vi "mini project.vi"() -> ()   [LabVIEW 2013]
panel:
  out "resulting string":string
  out "x":u8
  out "unsigned byte array":u8[](array[numeric])
  in  "String":string
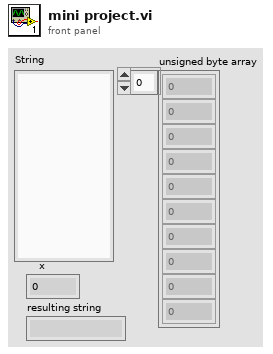
[diagram p1: front panel]
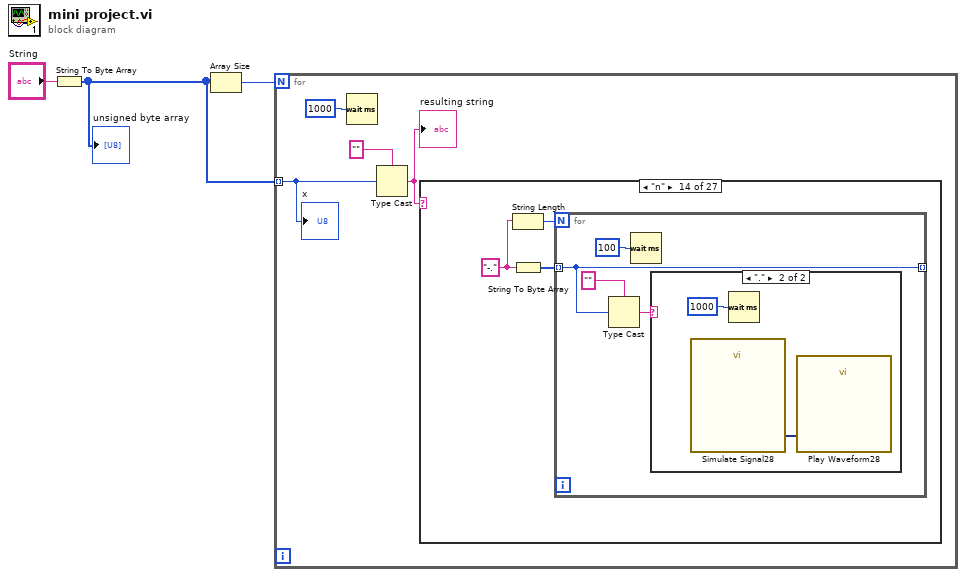
[diagram p0: block diagram]
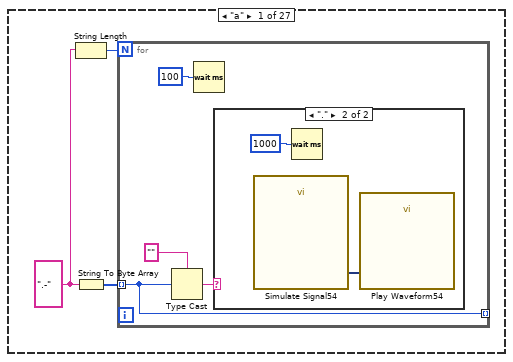
[diagram p2: hidden frame]
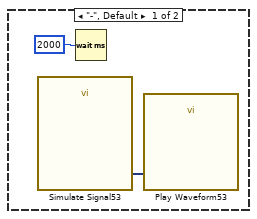
[diagram p3: hidden frame]
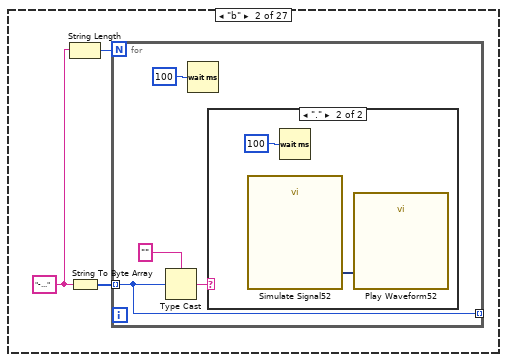
[diagram p4: hidden frame]
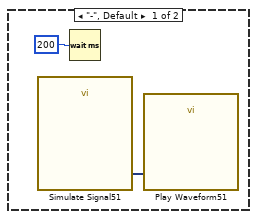
[diagram p5: hidden frame]
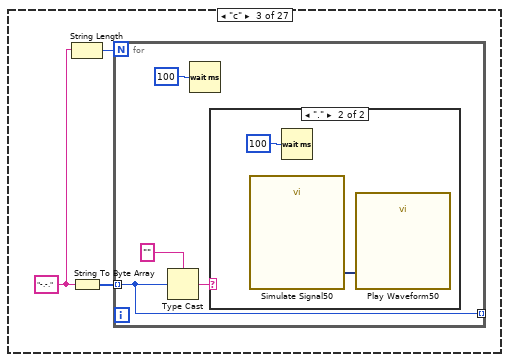
[diagram p6: hidden frame]
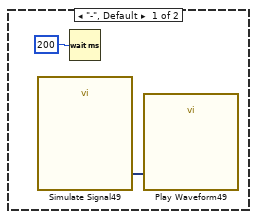
[diagram p7: hidden frame]
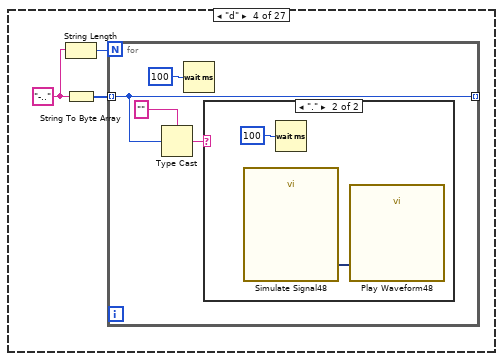
[diagram p8: hidden frame]
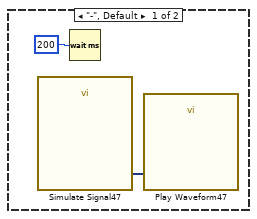
[diagram p9: hidden frame]
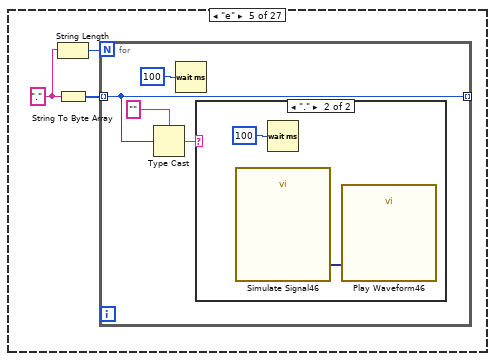
[diagram p10: hidden frame]
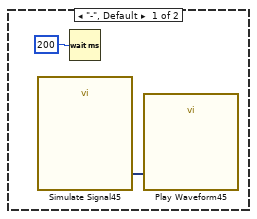
[diagram p11: hidden frame]
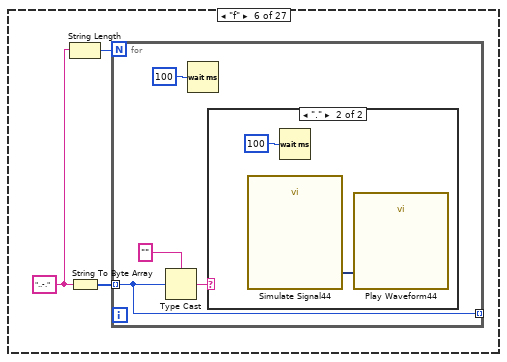
[diagram p12: hidden frame]
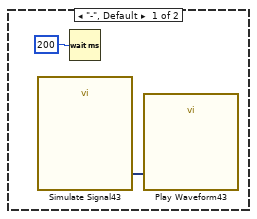
[diagram p13: hidden frame]
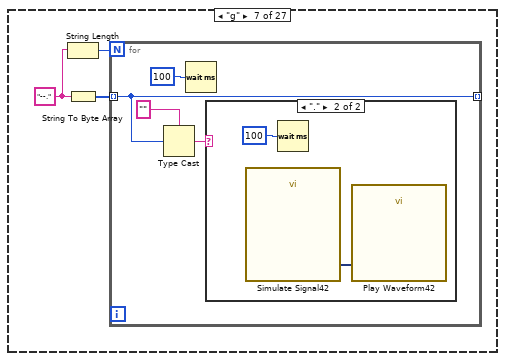
[diagram p14: hidden frame]
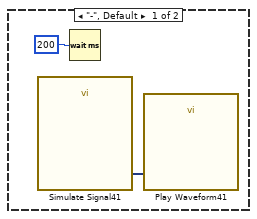
[diagram p15: hidden frame]
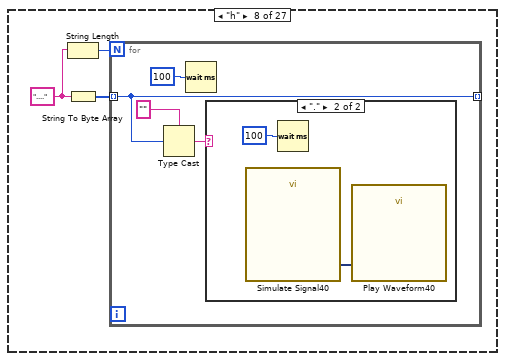
[diagram p16: hidden frame]
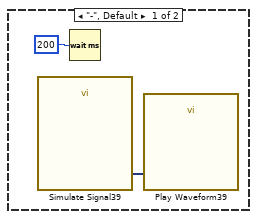
[diagram p17: hidden frame]
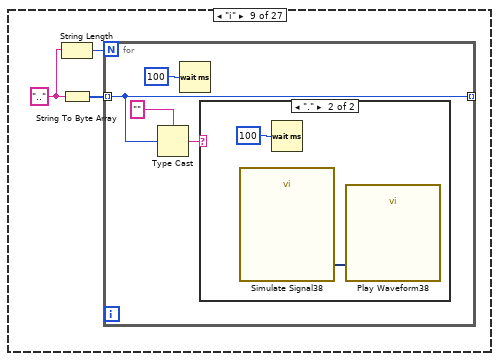
[diagram p18: hidden frame]
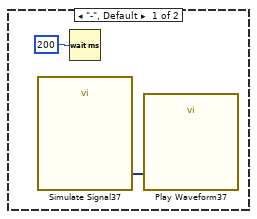
[diagram p19: hidden frame]
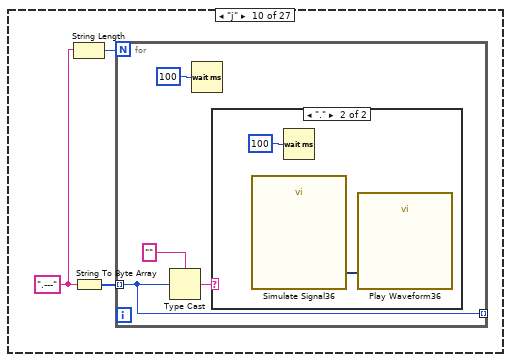
[diagram p20: hidden frame]
diagram:
  n1 = String To Byte Array(string="String") -> (unsigned byte array=w2:u8[])
  "unsigned byte array" <- w2
  n2 = Array Size(array=w2) -> (size(s)=w3:i32)
  n3 = for {
    N: w3 -> [_]
    tunnel: w2 -> [w7] mode=indexing
    n4 = Wait (ms)(milliseconds to wait=u32 1000) -> ()  [unwired: 1 out]
    n5 = Type Cast(type="", x=w7) -> (*(type *) &x=w5:string)
    "resulting string" <- w5
    n6 = case shown="\"n\"" w5 {
      frame "a" {
        w8 = ".-"
        n7 = String Length(string=w8) -> (length=w10:i32)
        n8 = String To Byte Array(string=w8) -> (unsigned byte array=w9:u8[])
        n9 = for {
          N: w10 -> [_]
          tunnel: [w13] -> _ mode=indexing
          tunnel: w9 -> [w13] mode=indexing
          n10 = Type Cast(type="", x=w13) -> (*(type *) &x=w11:string)
          n11 = Wait (ms)(milliseconds to wait=u32 100) -> ()  [unwired: 1 out]
          n12 = case shown="\".\"" w11 {
            frame "-", Default {
              n13 = call "Simulate Signal53"() -> ("Sine"=w16:dynamicdata)  [unwired: 14 in, 1 out]
              n14 = Wait (ms)(milliseconds to wait=u32 2000) -> ()  [unwired: 1 out]
              n15 = call "Play Waveform53"("Data"=w16) -> ()  [unwired: 18 in, 1 out]
            }
            frame "." {
              n16 = call "Simulate Signal54"() -> ("Sine"=w17:dynamicdata)  [unwired: 14 in, 1 out]
              n17 = Wait (ms)(milliseconds to wait=u32 1000) -> ()  [unwired: 1 out]
              n18 = call "Play Waveform54"("Data"=w17) -> ()  [unwired: 18 in, 1 out]
            }
          }
        }
      }
      frame "b" {
        w19 = "-..."
        n19 = String Length(string=w19) -> (length=w21:i32)
        n20 = String To Byte Array(string=w19) -> (unsigned byte array=w20:u8[])
        n21 = for {
          N: w21 -> [_]
          tunnel: [w24] -> _ mode=indexing
          tunnel: w20 -> [w24] mode=indexing
          n22 = Type Cast(type="", x=w24) -> (*(type *) &x=w22:string)
          n23 = Wait (ms)(milliseconds to wait=u32 100) -> ()  [unwired: 1 out]
          n24 = case shown="\".\"" w22 {
            frame "-", Default {
              n25 = call "Simulate Signal51"() -> ("Sine"=w27:dynamicdata)  [unwired: 14 in, 1 out]
              n26 = Wait (ms)(milliseconds to wait=u32 200) -> ()  [unwired: 1 out]
              n27 = call "Play Waveform51"("Data"=w27) -> ()  [unwired: 18 in, 1 out]
            }
            frame "." {
              n28 = call "Simulate Signal52"() -> ("Sine"=w28:dynamicdata)  [unwired: 14 in, 1 out]
              n29 = Wait (ms)(milliseconds to wait=u32 100) -> ()  [unwired: 1 out]
              n30 = call "Play Waveform52"("Data"=w28) -> ()  [unwired: 18 in, 1 out]
            }
          }
        }
      }
      frame "c" {
        w30 = "-.-."
        n31 = String Length(string=w30) -> (length=w32:i32)
        n32 = String To Byte Array(string=w30) -> (unsigned byte array=w31:u8[])
        n33 = for {
          N: w32 -> [_]
          tunnel: [w35] -> _ mode=indexing
          tunnel: w31 -> [w35] mode=indexing
          n34 = Type Cast(type="", x=w35) -> (*(type *) &x=w33:string)
          n35 = Wait (ms)(milliseconds to wait=u32 100) -> ()  [unwired: 1 out]
          n36 = case shown="\".\"" w33 {
            frame "-", Default {
              n37 = call "Simulate Signal49"() -> ("Sine"=w38:dynamicdata)  [unwired: 14 in, 1 out]
              n38 = Wait (ms)(milliseconds to wait=u32 200) -> ()  [unwired: 1 out]
              n39 = call "Play Waveform49"("Data"=w38) -> ()  [unwired: 18 in, 1 out]
            }
            frame "." {
              n40 = call "Simulate Signal50"() -> ("Sine"=w39:dynamicdata)  [unwired: 14 in, 1 out]
              n41 = Wait (ms)(milliseconds to wait=u32 100) -> ()  [unwired: 1 out]
              n42 = call "Play Waveform50"("Data"=w39) -> ()  [unwired: 18 in, 1 out]
            }
          }
        }
      }
      frame "d" {
        w41 = "-.."
        n43 = String Length(string=w41) -> (length=w43:i32)
        n44 = String To Byte Array(string=w41) -> (unsigned byte array=w42:u8[])
        n45 = for {
          N: w43 -> [_]
          tunnel: [w46] -> _ mode=indexing
          tunnel: w42 -> [w46] mode=indexing
          n46 = Type Cast(type="", x=w46) -> (*(type *) &x=w44:string)
          n47 = Wait (ms)(milliseconds to wait=u32 100) -> ()  [unwired: 1 out]
          n48 = case shown="\".\"" w44 {
            frame "-", Default {
              n49 = call "Simulate Signal47"() -> ("Sine"=w49:dynamicdata)  [unwired: 14 in, 1 out]
              n50 = Wait (ms)(milliseconds to wait=u32 200) -> ()  [unwired: 1 out]
              n51 = call "Play Waveform47"("Data"=w49) -> ()  [unwired: 18 in, 1 out]
            }
            frame "." {
              n52 = call "Simulate Signal48"() -> ("Sine"=w50:dynamicdata)  [unwired: 14 in, 1 out]
              n53 = Wait (ms)(milliseconds to wait=u32 100) -> ()  [unwired: 1 out]
              n54 = call "Play Waveform48"("Data"=w50) -> ()  [unwired: 18 in, 1 out]
            }
          }
        }
      }
      frame "e" {
        w52 = "."
        n55 = String Length(string=w52) -> (length=w54:i32)
        n56 = String To Byte Array(string=w52) -> (unsigned byte array=w53:u8[])
        n57 = for {
          N: w54 -> [_]
          tunnel: [w57] -> _ mode=indexing
          tunnel: w53 -> [w57] mode=indexing
          n58 = Type Cast(type="", x=w57) -> (*(type *) &x=w55:string)
          n59 = Wait (ms)(milliseconds to wait=u32 100) -> ()  [unwired: 1 out]
          n60 = case shown="\".\"" w55 {
            frame "-", Default {
              n61 = call "Simulate Signal45"() -> ("Sine"=w60:dynamicdata)  [unwired: 14 in, 1 out]
              n62 = Wait (ms)(milliseconds to wait=u32 200) -> ()  [unwired: 1 out]
              n63 = call "Play Waveform45"("Data"=w60) -> ()  [unwired: 18 in, 1 out]
            }
            frame "." {
              n64 = call "Simulate Signal46"() -> ("Sine"=w61:dynamicdata)  [unwired: 14 in, 1 out]
              n65 = Wait (ms)(milliseconds to wait=u32 100) -> ()  [unwired: 1 out]
              n66 = call "Play Waveform46"("Data"=w61) -> ()  [unwired: 18 in, 1 out]
            }
          }
        }
      }
      frame "f" {
        w63 = "..-."
        n67 = String Length(string=w63) -> (length=w65:i32)
        n68 = String To Byte Array(string=w63) -> (unsigned byte array=w64:u8[])
        n69 = for {
          N: w65 -> [_]
          tunnel: [w68] -> _ mode=indexing
          tunnel: w64 -> [w68] mode=indexing
          n70 = Type Cast(type="", x=w68) -> (*(type *) &x=w66:string)
          n71 = Wait (ms)(milliseconds to wait=u32 100) -> ()  [unwired: 1 out]
          n72 = case shown="\".\"" w66 {
            frame "-", Default {
              n73 = call "Simulate Signal43"() -> ("Sine"=w71:dynamicdata)  [unwired: 14 in, 1 out]
              n74 = Wait (ms)(milliseconds to wait=u32 200) -> ()  [unwired: 1 out]
              n75 = call "Play Waveform43"("Data"=w71) -> ()  [unwired: 18 in, 1 out]
            }
            frame "." {
              n76 = call "Simulate Signal44"() -> ("Sine"=w72:dynamicdata)  [unwired: 14 in, 1 out]
              n77 = Wait (ms)(milliseconds to wait=u32 100) -> ()  [unwired: 1 out]
              n78 = call "Play Waveform44"("Data"=w72) -> ()  [unwired: 18 in, 1 out]
            }
          }
        }
      }
      frame "g" {
        w74 = "--."
        n79 = String Length(string=w74) -> (length=w76:i32)
        n80 = String To Byte Array(string=w74) -> (unsigned byte array=w75:u8[])
        n81 = for {
          N: w76 -> [_]
          tunnel: [w79] -> _ mode=indexing
          tunnel: w75 -> [w79] mode=indexing
          n82 = Type Cast(type="", x=w79) -> (*(type *) &x=w77:string)
          n83 = Wait (ms)(milliseconds to wait=u32 100) -> ()  [unwired: 1 out]
          n84 = case shown="\".\"" w77 {
            frame "-", Default {
              n85 = call "Simulate Signal41"() -> ("Sine"=w82:dynamicdata)  [unwired: 14 in, 1 out]
              n86 = Wait (ms)(milliseconds to wait=u32 200) -> ()  [unwired: 1 out]
              n87 = call "Play Waveform41"("Data"=w82) -> ()  [unwired: 18 in, 1 out]
            }
            frame "." {
              n88 = call "Simulate Signal42"() -> ("Sine"=w83:dynamicdata)  [unwired: 14 in, 1 out]
              n89 = Wait (ms)(milliseconds to wait=u32 100) -> ()  [unwired: 1 out]
              n90 = call "Play Waveform42"("Data"=w83) -> ()  [unwired: 18 in, 1 out]
            }
          }
        }
      }
      frame "h" {
        w85 = "...."
        n91 = String Length(string=w85) -> (length=w87:i32)
        n92 = String To Byte Array(string=w85) -> (unsigned byte array=w86:u8[])
        n93 = for {
          N: w87 -> [_]
          tunnel: [w90] -> _ mode=indexing
          tunnel: w86 -> [w90] mode=indexing
          n94 = Type Cast(type="", x=w90) -> (*(type *) &x=w88:string)
          n95 = Wait (ms)(milliseconds to wait=u32 100) -> ()  [unwired: 1 out]
          n96 = case shown="\".\"" w88 {
            frame "-", Default {
              n97 = call "Simulate Signal39"() -> ("Sine"=w93:dynamicdata)  [unwired: 14 in, 1 out]
              n98 = Wait (ms)(milliseconds to wait=u32 200) -> ()  [unwired: 1 out]
              n99 = call "Play Waveform39"("Data"=w93) -> ()  [unwired: 18 in, 1 out]
            }
            frame "." {
              n100 = call "Simulate Signal40"() -> ("Sine"=w94:dynamicdata)  [unwired: 14 in, 1 out]
              n101 = Wait (ms)(milliseconds to wait=u32 100) -> ()  [unwired: 1 out]
              n102 = call "Play Waveform40"("Data"=w94) -> ()  [unwired: 18 in, 1 out]
            }
          }
        }
      }
      frame "i" {
        w96 = ".."
        n103 = String Length(string=w96) -> (length=w98:i32)
        n104 = String To Byte Array(string=w96) -> (unsigned byte array=w97:u8[])
        n105 = for {
          N: w98 -> [_]
          tunnel: [w101] -> _ mode=indexing
          tunnel: w97 -> [w101] mode=indexing
          n106 = Type Cast(type="", x=w101) -> (*(type *) &x=w99:string)
          n107 = Wait (ms)(milliseconds to wait=u32 100) -> ()  [unwired: 1 out]
          n108 = case shown="\".\"" w99 {
            frame "-", Default {
              n109 = call "Simulate Signal37"() -> ("Sine"=w104:dynamicdata)  [unwired: 14 in, 1 out]
              n110 = Wait (ms)(milliseconds to wait=u32 200) -> ()  [unwired: 1 out]
              n111 = call "Play Waveform37"("Data"=w104) -> ()  [unwired: 18 in, 1 out]
            }
            frame "." {
              n112 = call "Simulate Signal38"() -> ("Sine"=w105:dynamicdata)  [unwired: 14 in, 1 out]
              n113 = Wait (ms)(milliseconds to wait=u32 100) -> ()  [unwired: 1 out]
              n114 = call "Play Waveform38"("Data"=w105) -> ()  [unwired: 18 in, 1 out]
            }
          }
        }
      }
      frame "j" {
        w107 = ".---"
        n115 = String Length(string=w107) -> (length=w109:i32)
        n116 = String To Byte Array(string=w107) -> (unsigned byte array=w108:u8[])
        n117 = for {
          N: w109 -> [_]
          tunnel: [w112] -> _ mode=indexing
          tunnel: w108 -> [w112] mode=indexing
          n118 = Type Cast(type="", x=w112) -> (*(type *) &x=w110:string)
          n119 = Wait (ms)(milliseconds to wait=u32 100) -> ()  [unwired: 1 out]
          n120 = case shown="\".\"" w110 {
            frame "-", Default {
              n121 = call "Simulate Signal35"() -> ("Sine"=w115:dynamicdata)  [unwired: 14 in, 1 out]
              n122 = Wait (ms)(milliseconds to wait=u32 200) -> ()  [unwired: 1 out]
              n123 = call "Play Waveform35"("Data"=w115) -> ()  [unwired: 18 in, 1 out]
            }
            frame "." {
              n124 = call "Simulate Signal36"() -> ("Sine"=w116:dynamicdata)  [unwired: 14 in, 1 out]
              n125 = Wait (ms)(milliseconds to wait=u32 100) -> ()  [unwired: 1 out]
              n126 = call "Play Waveform36"("Data"=w116) -> ()  [unwired: 18 in, 1 out]
            }
          }
        }
      }
      frame "k" {
        w118 = "-.-"
        n127 = String Length(string=w118) -> (length=w120:i32)
        n128 = String To Byte Array(string=w118) -> (unsigned byte array=w119:u8[])
        n129 = for {
          N: w120 -> [_]
          tunnel: [w123] -> _ mode=indexing
          tunnel: w119 -> [w123] mode=indexing
          n130 = Type Cast(type="", x=w123) -> (*(type *) &x=w121:string)
          n131 = Wait (ms)(milliseconds to wait=u32 100) -> ()  [unwired: 1 out]
          n132 = case shown="\".\"" w121 {
            frame "-", Default {
              n133 = call "Simulate Signal33"() -> ("Sine"=w126:dynamicdata)  [unwired: 14 in, 1 out]
              n134 = Wait (ms)(milliseconds to wait=u32 200) -> ()  [unwired: 1 out]
              n135 = call "Play Waveform33"("Data"=w126) -> ()  [unwired: 18 in, 1 out]
            }
            frame "." {
              n136 = call "Simulate Signal34"() -> ("Sine"=w127:dynamicdata)  [unwired: 14 in, 1 out]
              n137 = Wait (ms)(milliseconds to wait=u32 100) -> ()  [unwired: 1 out]
              n138 = call "Play Waveform34"("Data"=w127) -> ()  [unwired: 18 in, 1 out]
            }
          }
        }
      }
      frame "l" {
        w129 = ".-.."
        n139 = String Length(string=w129) -> (length=w131:i32)
        n140 = String To Byte Array(string=w129) -> (unsigned byte array=w130:u8[])
        n141 = for {
          N: w131 -> [_]
          tunnel: [w134] -> _ mode=indexing
          tunnel: w130 -> [w134] mode=indexing
          n142 = Type Cast(type="", x=w134) -> (*(type *) &x=w132:string)
          n143 = Wait (ms)(milliseconds to wait=u32 100) -> ()  [unwired: 1 out]
          n144 = case shown="\".\"" w132 {
            frame "-", Default {
              n145 = call "Simulate Signal31"() -> ("Sine"=w137:dynamicdata)  [unwired: 14 in, 1 out]
              n146 = Wait (ms)(milliseconds to wait=u32 200) -> ()  [unwired: 1 out]
              n147 = call "Play Waveform31"("Data"=w137) -> ()  [unwired: 18 in, 1 out]
            }
            frame "." {
              n148 = call "Simulate Signal32"() -> ("Sine"=w138:dynamicdata)  [unwired: 14 in, 1 out]
              n149 = Wait (ms)(milliseconds to wait=u32 100) -> ()  [unwired: 1 out]
              n150 = call "Play Waveform32"("Data"=w138) -> ()  [unwired: 18 in, 1 out]
            }
          }
        }
      }
      frame "m" {
        w140 = "--"
        n151 = String Length(string=w140) -> (length=w142:i32)
        n152 = String To Byte Array(string=w140) -> (unsigned byte array=w141:u8[])
        n153 = for {
          N: w142 -> [_]
          tunnel: [w145] -> _ mode=indexing
          tunnel: w141 -> [w145] mode=indexing
          n154 = Type Cast(type="", x=w145) -> (*(type *) &x=w143:string)
          n155 = Wait (ms)(milliseconds to wait=u32 100) -> ()  [unwired: 1 out]
          n156 = case shown="\".\"" w143 {
            frame "-", Default {
              n157 = call "Simulate Signal29"() -> ("Sine"=w148:dynamicdata)  [unwired: 14 in, 1 out]
              n158 = Wait (ms)(milliseconds to wait=u32 200) -> ()  [unwired: 1 out]
              n159 = call "Play Waveform29"("Data"=w148) -> ()  [unwired: 18 in, 1 out]
            }
            frame "." {
              n160 = call "Simulate Signal30"() -> ("Sine"=w149:dynamicdata)  [unwired: 14 in, 1 out]
              n161 = Wait (ms)(milliseconds to wait=u32 100) -> ()  [unwired: 1 out]
              n162 = call "Play Waveform30"("Data"=w149) -> ()  [unwired: 18 in, 1 out]
            }
          }
        }
      }
      frame "n" {
        w151 = "-."
        n163 = String Length(string=w151) -> (length=w153:i32)
        n164 = String To Byte Array(string=w151) -> (unsigned byte array=w152:u8[])
        n165 = for {
          N: w153 -> [_]
          tunnel: [w156] -> _ mode=indexing
          tunnel: w152 -> [w156] mode=indexing
          n166 = Type Cast(type="", x=w156) -> (*(type *) &x=w154:string)
          n167 = Wait (ms)(milliseconds to wait=u32 100) -> ()  [unwired: 1 out]
          n168 = case shown="\".\"" w154 {
            frame "-", Default {
              n169 = call "Simulate Signal27"() -> ("Sine"=w159:dynamicdata)  [unwired: 14 in, 1 out]
              n170 = Wait (ms)(milliseconds to wait=u32 2000) -> ()  [unwired: 1 out]
              n171 = call "Play Waveform27"("Data"=w159) -> ()  [unwired: 18 in, 1 out]
            }
            frame "." {
              n172 = call "Simulate Signal28"() -> ("Sine"=w160:dynamicdata)  [unwired: 14 in, 1 out]
              n173 = Wait (ms)(milliseconds to wait=u32 1000) -> ()  [unwired: 1 out]
              n174 = call "Play Waveform28"("Data"=w160) -> ()  [unwired: 18 in, 1 out]
            }
          }
        }
      }
      frame "o" {
        w162 = "---"
        n175 = String Length(string=w162) -> (length=w164:i32)
        n176 = String To Byte Array(string=w162) -> (unsigned byte array=w163:u8[])
        n177 = for {
          N: w164 -> [_]
          tunnel: [w167] -> _ mode=indexing
          tunnel: w163 -> [w167] mode=indexing
          n178 = Type Cast(type="", x=w167) -> (*(type *) &x=w165:string)
          n179 = Wait (ms)(milliseconds to wait=u32 100) -> ()  [unwired: 1 out]
          n180 = case shown="\".\"" w165 {
            frame "-", Default {
              n181 = call "Simulate Signal25"() -> ("Sine"=w170:dynamicdata)  [unwired: 14 in, 1 out]
              n182 = Wait (ms)(milliseconds to wait=u32 200) -> ()  [unwired: 1 out]
              n183 = call "Play Waveform25"("Data"=w170) -> ()  [unwired: 18 in, 1 out]
            }
            frame "." {
              n184 = call "Simulate Signal26"() -> ("Sine"=w171:dynamicdata)  [unwired: 14 in, 1 out]
              n185 = Wait (ms)(milliseconds to wait=u32 100) -> ()  [unwired: 1 out]
              n186 = call "Play Waveform26"("Data"=w171) -> ()  [unwired: 18 in, 1 out]
            }
          }
        }
      }
      frame "p" {
        w173 = ".--."
        n187 = String Length(string=w173) -> (length=w175:i32)
        n188 = String To Byte Array(string=w173) -> (unsigned byte array=w174:u8[])
        n189 = for {
          N: w175 -> [_]
          tunnel: [w178] -> _ mode=indexing
          tunnel: w174 -> [w178] mode=indexing
          n190 = Type Cast(type="", x=w178) -> (*(type *) &x=w176:string)
          n191 = Wait (ms)(milliseconds to wait=u32 100) -> ()  [unwired: 1 out]
          n192 = case shown="\".\"" w176 {
            frame "-", Default {
              n193 = call "Simulate Signal23"() -> ("Sine"=w181:dynamicdata)  [unwired: 14 in, 1 out]
              n194 = Wait (ms)(milliseconds to wait=u32 200) -> ()  [unwired: 1 out]
              n195 = call "Play Waveform23"("Data"=w181) -> ()  [unwired: 18 in, 1 out]
            }
            frame "." {
              n196 = call "Simulate Signal24"() -> ("Sine"=w182:dynamicdata)  [unwired: 14 in, 1 out]
              n197 = Wait (ms)(milliseconds to wait=u32 100) -> ()  [unwired: 1 out]
              n198 = call "Play Waveform24"("Data"=w182) -> ()  [unwired: 18 in, 1 out]
            }
          }
        }
      }
      frame "q" {
        w184 = "--.-"
        n199 = String Length(string=w184) -> (length=w186:i32)
        n200 = String To Byte Array(string=w184) -> (unsigned byte array=w185:u8[])
        n201 = for {
          N: w186 -> [_]
          tunnel: [w189] -> _ mode=indexing
          tunnel: w185 -> [w189] mode=indexing
          n202 = Type Cast(type="", x=w189) -> (*(type *) &x=w187:string)
          n203 = Wait (ms)(milliseconds to wait=u32 100) -> ()  [unwired: 1 out]
          n204 = case shown="\".\"" w187 {
            frame "-", Default {
              n205 = call "Simulate Signal21"() -> ("Sine"=w192:dynamicdata)  [unwired: 14 in, 1 out]
              n206 = Wait (ms)(milliseconds to wait=u32 200) -> ()  [unwired: 1 out]
              n207 = call "Play Waveform21"("Data"=w192) -> ()  [unwired: 18 in, 1 out]
            }
            frame "." {
              n208 = call "Simulate Signal22"() -> ("Sine"=w193:dynamicdata)  [unwired: 14 in, 1 out]
              n209 = Wait (ms)(milliseconds to wait=u32 100) -> ()  [unwired: 1 out]
              n210 = call "Play Waveform22"("Data"=w193) -> ()  [unwired: 18 in, 1 out]
            }
          }
        }
      }
      frame "r" {
        w195 = ".-."
        n211 = String Length(string=w195) -> (length=w197:i32)
        n212 = String To Byte Array(string=w195) -> (unsigned byte array=w196:u8[])
        n213 = for {
          N: w197 -> [_]
          tunnel: [w200] -> _ mode=indexing
          tunnel: w196 -> [w200] mode=indexing
          n214 = Type Cast(type="", x=w200) -> (*(type *) &x=w198:string)
          n215 = Wait (ms)(milliseconds to wait=u32 100) -> ()  [unwired: 1 out]
          n216 = case shown="\".\"" w198 {
            frame "-", Default {
              n217 = call "Simulate Signal19"() -> ("Sine"=w203:dynamicdata)  [unwired: 14 in, 1 out]
              n218 = Wait (ms)(milliseconds to wait=u32 200) -> ()  [unwired: 1 out]
              n219 = call "Play Waveform19"("Data"=w203) -> ()  [unwired: 18 in, 1 out]
            }
            frame "." {
              n220 = call "Simulate Signal20"() -> ("Sine"=w204:dynamicdata)  [unwired: 14 in, 1 out]
              n221 = Wait (ms)(milliseconds to wait=u32 100) -> ()  [unwired: 1 out]
              n222 = call "Play Waveform20"("Data"=w204) -> ()  [unwired: 18 in, 1 out]
            }
          }
        }
      }
      frame "s" {
        w206 = "..."
        n223 = String Length(string=w206) -> (length=w208:i32)
        n224 = String To Byte Array(string=w206) -> (unsigned byte array=w207:u8[])
        n225 = for {
          N: w208 -> [_]
          tunnel: [w211] -> _ mode=indexing
          tunnel: w207 -> [w211] mode=indexing
          n226 = Type Cast(type="", x=w211) -> (*(type *) &x=w209:string)
          n227 = Wait (ms)(milliseconds to wait=u32 100) -> ()  [unwired: 1 out]
          n228 = case shown="\".\"" w209 {
            frame "-", Default {
              n229 = call "Simulate Signal17"() -> ("Sine"=w214:dynamicdata)  [unwired: 14 in, 1 out]
              n230 = Wait (ms)(milliseconds to wait=u32 200) -> ()  [unwired: 1 out]
              n231 = call "Play Waveform17"("Data"=w214) -> ()  [unwired: 18 in, 1 out]
            }
            frame "." {
              n232 = call "Simulate Signal18"() -> ("Sine"=w215:dynamicdata)  [unwired: 14 in, 1 out]
              n233 = Wait (ms)(milliseconds to wait=u32 100) -> ()  [unwired: 1 out]
              n234 = call "Play Waveform18"("Data"=w215) -> ()  [unwired: 18 in, 1 out]
            }
          }
        }
      }
      frame "t" {
        w217 = "-"
        n235 = String Length(string=w217) -> (length=w219:i32)
        n236 = String To Byte Array(string=w217) -> (unsigned byte array=w218:u8[])
        n237 = for {
          N: w219 -> [_]
          tunnel: [w222] -> _ mode=indexing
          tunnel: w218 -> [w222] mode=indexing
          n238 = Type Cast(type="", x=w222) -> (*(type *) &x=w220:string)
          n239 = Wait (ms)(milliseconds to wait=u32 100) -> ()  [unwired: 1 out]
          n240 = case shown="\".\"" w220 {
            frame "-", Default {
              n241 = call "Simulate Signal15"() -> ("Sine"=w225:dynamicdata)  [unwired: 14 in, 1 out]
              n242 = Wait (ms)(milliseconds to wait=u32 200) -> ()  [unwired: 1 out]
              n243 = call "Play Waveform15"("Data"=w225) -> ()  [unwired: 18 in, 1 out]
            }
            frame "." {
              n244 = call "Simulate Signal16"() -> ("Sine"=w226:dynamicdata)  [unwired: 14 in, 1 out]
              n245 = Wait (ms)(milliseconds to wait=u32 100) -> ()  [unwired: 1 out]
              n246 = call "Play Waveform16"("Data"=w226) -> ()  [unwired: 18 in, 1 out]
            }
          }
        }
      }
      frame "u" {
        w228 = "..-"
        n247 = String Length(string=w228) -> (length=w230:i32)
        n248 = String To Byte Array(string=w228) -> (unsigned byte array=w229:u8[])
        n249 = for {
          N: w230 -> [_]
          tunnel: [w233] -> _ mode=indexing
          tunnel: w229 -> [w233] mode=indexing
          n250 = Type Cast(type="", x=w233) -> (*(type *) &x=w231:string)
          n251 = Wait (ms)(milliseconds to wait=u32 100) -> ()  [unwired: 1 out]
          n252 = case shown="\".\"" w231 {
            frame "-", Default {
              n253 = call "Simulate Signal13"() -> ("Sine"=w236:dynamicdata)  [unwired: 14 in, 1 out]
              n254 = Wait (ms)(milliseconds to wait=u32 200) -> ()  [unwired: 1 out]
              n255 = call "Play Waveform13"("Data"=w236) -> ()  [unwired: 18 in, 1 out]
            }
            frame "." {
              n256 = call "Simulate Signal14"() -> ("Sine"=w237:dynamicdata)  [unwired: 14 in, 1 out]
              n257 = Wait (ms)(milliseconds to wait=u32 100) -> ()  [unwired: 1 out]
              n258 = call "Play Waveform14"("Data"=w237) -> ()  [unwired: 18 in, 1 out]
            }
          }
        }
      }
      frame "v" {
        w239 = "...-"
        n259 = String Length(string=w239) -> (length=w241:i32)
        n260 = String To Byte Array(string=w239) -> (unsigned byte array=w240:u8[])
        n261 = for {
          N: w241 -> [_]
          tunnel: [w244] -> _ mode=indexing
          tunnel: w240 -> [w244] mode=indexing
          n262 = Type Cast(type="", x=w244) -> (*(type *) &x=w242:string)
          n263 = Wait (ms)(milliseconds to wait=u32 100) -> ()  [unwired: 1 out]
          n264 = case shown="\".\"" w242 {
            frame "-", Default {
              n265 = call "Simulate Signal11"() -> ("Sine"=w247:dynamicdata)  [unwired: 14 in, 1 out]
              n266 = Wait (ms)(milliseconds to wait=u32 200) -> ()  [unwired: 1 out]
              n267 = call "Play Waveform11"("Data"=w247) -> ()  [unwired: 18 in, 1 out]
            }
            frame "." {
              n268 = call "Simulate Signal12"() -> ("Sine"=w248:dynamicdata)  [unwired: 14 in, 1 out]
              n269 = Wait (ms)(milliseconds to wait=u32 100) -> ()  [unwired: 1 out]
              n270 = call "Play Waveform12"("Data"=w248) -> ()  [unwired: 18 in, 1 out]
            }
          }
        }
      }
      frame "w" {
        w250 = ".--"
        n271 = String Length(string=w250) -> (length=w252:i32)
        n272 = String To Byte Array(string=w250) -> (unsigned byte array=w251:u8[])
        n273 = for {
          N: w252 -> [_]
          tunnel: [w255] -> _ mode=indexing
          tunnel: w251 -> [w255] mode=indexing
          n274 = Type Cast(type="", x=w255) -> (*(type *) &x=w253:string)
          n275 = Wait (ms)(milliseconds to wait=u32 100) -> ()  [unwired: 1 out]
          n276 = case shown="\".\"" w253 {
            frame "-", Default {
              n277 = call "Simulate Signal9"() -> ("Sine"=w258:dynamicdata)  [unwired: 14 in, 1 out]
              n278 = Wait (ms)(milliseconds to wait=u32 200) -> ()  [unwired: 1 out]
              n279 = call "Play Waveform9"("Data"=w258) -> ()  [unwired: 18 in, 1 out]
            }
            frame "." {
              n280 = call "Simulate Signal10"() -> ("Sine"=w259:dynamicdata)  [unwired: 14 in, 1 out]
              n281 = Wait (ms)(milliseconds to wait=u32 100) -> ()  [unwired: 1 out]
              n282 = call "Play Waveform10"("Data"=w259) -> ()  [unwired: 18 in, 1 out]
            }
          }
        }
      }
      frame "x" {
        w261 = "-..-"
        n283 = String Length(string=w261) -> (length=w263:i32)
        n284 = String To Byte Array(string=w261) -> (unsigned byte array=w262:u8[])
        n285 = for {
          N: w263 -> [_]
          tunnel: [w266] -> _ mode=indexing
          tunnel: w262 -> [w266] mode=indexing
          n286 = Type Cast(type="", x=w266) -> (*(type *) &x=w264:string)
          n287 = Wait (ms)(milliseconds to wait=u32 100) -> ()  [unwired: 1 out]
          n288 = case shown="\".\"" w264 {
            frame "-", Default {
              n289 = call "Simulate Signal7"() -> ("Sine"=w269:dynamicdata)  [unwired: 14 in, 1 out]
              n290 = Wait (ms)(milliseconds to wait=u32 200) -> ()  [unwired: 1 out]
              n291 = call "Play Waveform7"("Data"=w269) -> ()  [unwired: 18 in, 1 out]
            }
            frame "." {
              n292 = call "Simulate Signal8"() -> ("Sine"=w270:dynamicdata)  [unwired: 14 in, 1 out]
              n293 = Wait (ms)(milliseconds to wait=u32 100) -> ()  [unwired: 1 out]
              n294 = call "Play Waveform8"("Data"=w270) -> ()  [unwired: 18 in, 1 out]
            }
          }
        }
      }
      frame "y" {
        w272 = "-.--"
        n295 = String Length(string=w272) -> (length=w274:i32)
        n296 = String To Byte Array(string=w272) -> (unsigned byte array=w273:u8[])
        n297 = for {
          N: w274 -> [_]
          tunnel: [w277] -> _ mode=indexing
          tunnel: w273 -> [w277] mode=indexing
          n298 = Type Cast(type="", x=w277) -> (*(type *) &x=w275:string)
          n299 = Wait (ms)(milliseconds to wait=u32 100) -> ()  [unwired: 1 out]
          n300 = case shown="\".\"" w275 {
            frame "-", Default {
              n301 = call "Simulate Signal5"() -> ("Sine"=w280:dynamicdata)  [unwired: 14 in, 1 out]
              n302 = Wait (ms)(milliseconds to wait=u32 200) -> ()  [unwired: 1 out]
              n303 = call "Play Waveform5"("Data"=w280) -> ()  [unwired: 18 in, 1 out]
            }
            frame "." {
              n304 = call "Simulate Signal6"() -> ("Sine"=w281:dynamicdata)  [unwired: 14 in, 1 out]
              n305 = Wait (ms)(milliseconds to wait=u32 100) -> ()  [unwired: 1 out]
              n306 = call "Play Waveform6"("Data"=w281) -> ()  [unwired: 18 in, 1 out]
            }
          }
        }
      }
      frame "z" {
        w284 = "--.."
        n307 = String Length(string=w284) -> (length=w285:i32)
        n308 = String To Byte Array(string=w284) -> (unsigned byte array=w283:u8[])
        n309 = for {
          N: w285 -> [_]
          tunnel: [w288] -> _ mode=indexing
          tunnel: w283 -> [w288] mode=indexing
          n310 = Type Cast(type="", x=w288) -> (*(type *) &x=w286:string)
          n311 = Wait (ms)(milliseconds to wait=u32 100) -> ()  [unwired: 1 out]
          n312 = case shown="\".\"" w286 {
            frame "-", Default {
              n313 = call "Simulate Signal3"() -> ("Sine"=w291:dynamicdata)  [unwired: 14 in, 1 out]
              n314 = Wait (ms)(milliseconds to wait=u32 200) -> ()  [unwired: 1 out]
              n315 = call "Play Waveform3"("Data"=w291) -> ()  [unwired: 18 in, 1 out]
            }
            frame "." {
              n316 = call "Simulate Signal"() -> ("Sine"=w292:dynamicdata)  [unwired: 14 in, 1 out]
              n317 = Wait (ms)(milliseconds to wait=u32 100) -> ()  [unwired: 1 out]
              n318 = call "Play Waveform"("Data"=w292) -> ()  [unwired: 18 in, 1 out]
            }
          }
        }
      }
      frame "NULL", Default {
      }
    }
    "x" <- w7
  }
